vi "Read Callback Refs.vi"(8 "error in (no error)":errorcluster, 11 "teststand-api in":refnum<class "teststand-api.lvclass">) -> (0 "error out":errorcluster, 2 "Callback Refs":T1, 3 "teststand-api out":refnum<class "teststand-api.lvclass">)   [LabVIEW 2014, in "teststand-api.lvlib" / "teststand-api.lvclass"]
uses:
  teststand-api.lvclass
  Callback References Argument--cluster.ctl
  teststand-api.lvclass/teststand-api.ctl
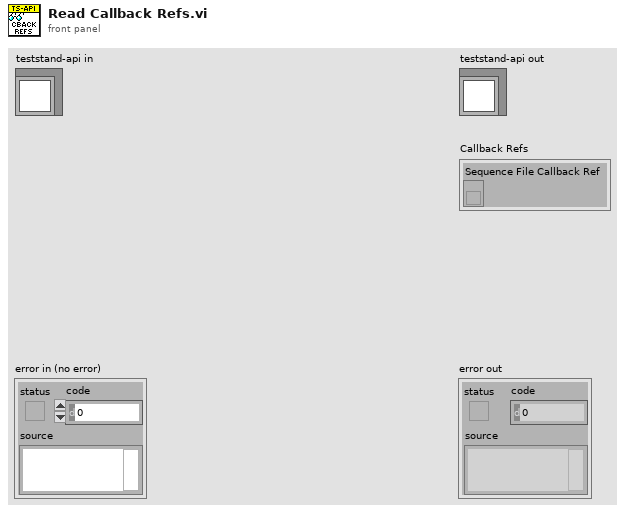
[diagram p1: front panel]
types:
  T1 = typedef "teststand-api.lvlib/teststand-api.lvclass/Callback References Argument--cluster.ctl" = cluster{"Sequence File Callback Ref":refnum<k27>}
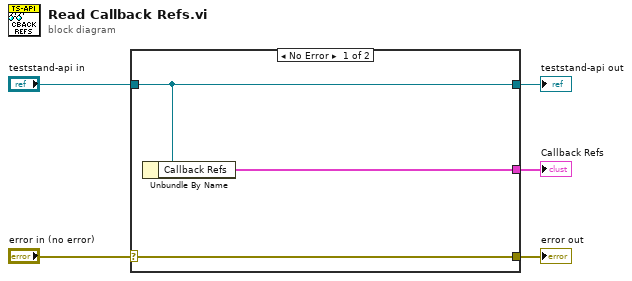
[diagram p0: block diagram]
diagram:
  n1 = case shown="No Error" "error in (no error)" {
    selector: "error in (no error)" -> [w8 w9]
    tunnel: [w8 w9] -> w4
    tunnel: [w7 w10] -> w2
    tunnel: "teststand-api in" -> [w7 w10]
    tunnel: [w6 _] -> w1
    frame No Error {
      n2 = Unbundle By Name(w7) -> ("Callback Refs"=w6:T1)
    }
    frame Error {
    }
  }
  "error out" <- w4
  "teststand-api out" <- w2
  "Callback Refs" <- w1
